vi "Configure Measurement Characteristics (AM Noise).vi"(0 "VISA resource name":refnum<visa-resource-name>, 1 "Measurement Quality (1: Normal)":u16(ring)=1 items=["Fast", "Normal"], 5 "Frequency Band (2: Band 4)":u16(ring)=2 items=["Band 2 (60E6 to 111E6 Hz)", "Band 3 (109E6 to 1.5E9 Hz)", "Band 4 (250E6 to 7E9 Hz)", "Band 5 (3E9 to 10E9 Hz)", "Band 6 (9E9 to 26.5E9 Hz)"], 7 "Enable Carrier Search (Disable)":bool, 9 "Manual Nominal Frequency (3E9 Hz)":dbl=3000000000.0 format="%^#_9g", 11 "error in (no error)":errorcluster, 12 "Enable Fast Measurement (Disable)":bool) -> (4 "VISA resource name out":refnum<visa-resource-name>, 15 "error out":errorcluster)   [LabVIEW 2011, in "Agilent E5052X.lvlib"]
doc: "Configures initial settings for AM Noise measurement.\n\n<b>Note:</b> \n\n1) AM Noise measurement is not available on the Agilent E5052A Signal Source Analyzer.\n\n2) This VI must be called first before calling \"Configure Measurement(AM Noise)\" VI."
uses:
  Agilent E5052X.lvlib
panel:
  # "Input Frequency Setting"
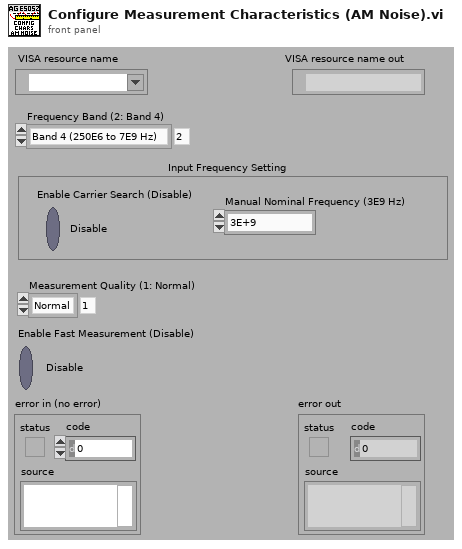
[diagram p1: front panel]
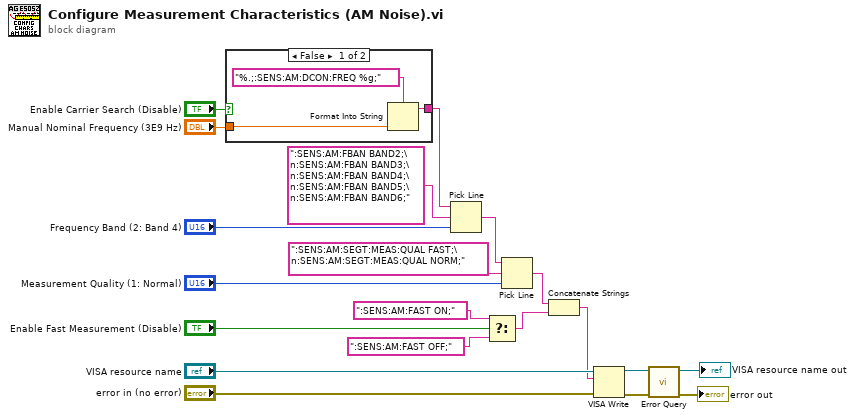
[diagram p0: block diagram]
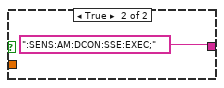
[diagram p2: hidden frame]
diagram:
  n1 = case shown="False" "Enable Carrier Search (Disable)" {
    tunnel: "Manual Nominal Frequency (3E9 Hz)" -> [w23 _]
    tunnel: [w21 ":SENS:AM:DCON:SSE:EXEC;" ("write buffer")] -> w5
    frame False {
      n2 = Format Into String(format string="%.;:SENS:AM:DCON:FREQ %g;", w23) -> (resulting string=w21:string)  [unwired: 2 in, 1 out]
    }
    frame True {
    }
  }
  n3 = Pick Line(string ("")=w5, multi-line string=":SENS:AM:FBAN BAND2;\n:SENS:AM:FBAN BAND3;\n:SENS:AM:FBAN BAND4;\n:SENS:AM:FBAN BAND5;\n:SENS:AM:FBAN BAND6;", line index="Frequency Band (2: Band 4)") -> (output string=w4:string)
  n4 = Select(t=":SENS:AM:FAST ON;", s="Enable Fast Measurement (Disable)", f=":SENS:AM:FAST OFF;") -> (s? t:f=w2:string)
  n5 = Pick Line(string ("")=w4, multi-line string=":SENS:AM:SEGT:MEAS:QUAL FAST;\n:SENS:AM:SEGT:MEAS:QUAL NORM;", line index="Measurement Quality (1: Normal)") -> (output string=w3:string)
  n6 = Concatenate Strings(w3, w2) -> (w1:string)
  n7 = VISA Write(VISA resource name="VISA resource name", write buffer=w1, error in (no error)="error in (no error)") -> (VISA resource name out=w20:refnum<visa-resource-name>, error out=w19:errorcluster)  [unwired: 1 out]
  n8 = call "Error Query.vi"("error in (no error)"=w19, "VISA resource name"=w20) -> ("error out"=→"error out":errorcluster, "VISA resource name out"=→"VISA resource name out":refnum<visa-resource-name>)  [unwired: 6 in, 2 out]
